vi "模式二.vi"(0 "Input Handle":cluster{"Session":u32, "Card number":u32}, 1 "文件夹路径":path caption="路径", 2 "设置":T1, 5 "error in":errorcluster {"code" format="%.0x"}) -> (14 "Output Handle":cluster{"Session":u32, "Card number":u32}, 19 "error out":errorcluster caption="error in")   [LabVIEW 2018]
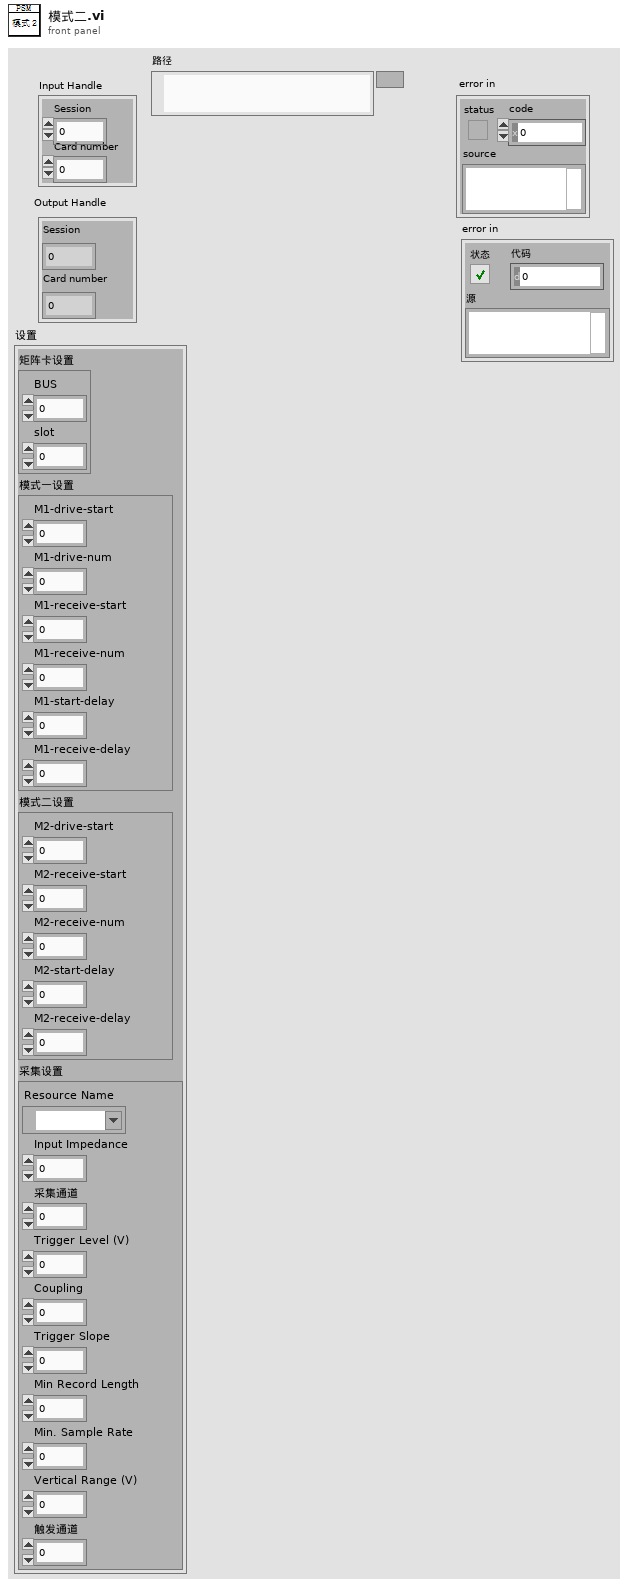
[diagram p1: front panel]
types:
  T1 = cluster{"矩阵卡设置":cluster{"BUS":u32, "slot":u32}, "模式一设置":cluster{"M1-drive-start":u32, "M1-drive-num":u32, "M1-receive-start":u32, "M1-receive-num":u32, "M1-start-delay":u32, "M1-receive-delay":u32}, "模式二设置":cluster{"M2-drive-start":u32, "M2-receive-start":u32, "M2-receive-num":u32, "M2-start-delay":u32, "M2-receive-delay":u32}, "采集设置":cluster{"Resource Name":refnum<k15>, "Input Impedance":u32, "采集通道":i32, "Trigger Level (V)":dbl, "Coupling":u16, "Trigger Slope":i32, "Min Record Length":i32, "Min. Sample Rate":dbl, "Vertical Range (V)":dbl, "触发通道":i32}}
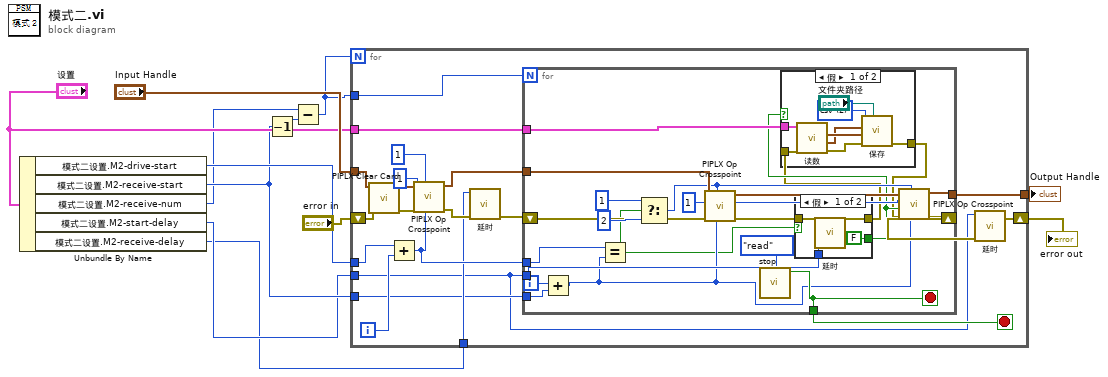
[diagram p0: block diagram]
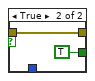
[diagram p3: hidden frame]
diagram:
  n1 = Unbundle By Name("设置") -> ("模式二设置.M2-drive-start"=w5:u32, "模式二设置.M2-receive-start"=w4:u32, "模式二设置.M2-receive-num"=w3:u32, "模式二设置.M2-start-delay"=w2:u32, "模式二设置.M2-receive-delay"=w1:u32)
  n2 = Decrement(x=w4) -> (x-1=w8:u32)
  n3 = Subtract(x=w3, y=w8) -> (x-y=w7:u32)
  n4 = for {
    N: w7 -> [_]
    tunnel: w7 -> [w33]
    tunnel: w5 -> [w30]
    tunnel: "Input Handle" -> [w28]
    tunnel: w2 -> [w14]
    shift-right: [w31] -> w9
    shift-left: "error in" -> [w27]
    tunnel: [w32] -> w10
    tunnel: w1 -> [w16]
    tunnel: w4 -> [w15]
    tunnel: "设置" -> [w13]
    i -> [w29]
    stop <- w20 stop-if-true
    n5 = call <instrlib>:"PIPLX Clear Card.vi"("error in"=w27, "Input Handle"=w28) -> ("error out"=w26:errorcluster, "Output Handle"=w25:cluster{"Session":u32, "Card number":u32})  [unwired: 8 in]
    n6 = Add(x=w30, y=w29) -> (x+y=w21:u32)
    n7 = call <instrlib>:"PIPLX Op Crosspoint.vi"("Column"=w21, "Row"=u32 1, "error in"=w26, "Output Subunit"=u32 1, "Input Handle"=w25) -> ("error out"=w19:errorcluster, "Output Handle"=w24:cluster{"Session":u32, "Card number":u32})  [unwired: 5 in]
    n8 = call "延时.vi"("error in (no error)"=w19, "延时（百毫秒）"=w16) -> ("error out"=w18:errorcluster)  [unwired: 9 in]
    n9 = for {
      N: w33 -> [_]
      tunnel: w21 -> [w53]
      tunnel: w24 -> [w52]
      tunnel: w14 -> [w50]
      shift-right: [w36] -> w17
      shift-left: w18 -> [w51]
      tunnel: [w46] -> w32
      tunnel: [w47] -> w20
      tunnel: w15 -> [w40]
      tunnel: w13 -> [w38]
      i -> [w42]
      stop <- w47 stop-if-true
      w44 = u32 1 ("Output Subunit")
      n10 = Add(x=w42, y=w40) -> (x+y=w41:u32)
      n11 = Equal?(x=w53, y=w41) -> (x = y?=w39:bool)
      n12 = Select(t=u32 1 ("Row"), s=w39, f=u32 2) -> (s? t:f=w43:u32)
      n13 = call <instrlib>:"PIPLX Op Crosspoint.vi"("Column"=w41, "Row"=w43, "error in"=w51, "Output Subunit"=w44, "Input Handle"=w52) -> ("error out"=w49:errorcluster, "Output Handle"=w45:cluster{"Session":u32, "Card number":u32})  [unwired: 5 in]
      n14 = call "stop.vi"("枚举"=enum16{"write", "read"}."read") -> ("停止"=w47:bool)  [unwired: 10 in]
      n15 = case shown="假" w39 {
        tunnel: w50 -> [w68 _]
        tunnel: w49 -> [w67 w70]
        tunnel: [w66 w70] -> w34
        tunnel: [FALSE ("Action") TRUE ("Action")] -> w37
        frame False {
          n16 = call "延时.vi"("error in (no error)"=w67, "延时（百毫秒）"=w68) -> ("error out"=w66:errorcluster)  [unwired: 9 in]
        }
        frame True {
        }
      }
      n17 = case shown="假" w37 {
        tunnel: w34 -> [w56 w64]
        tunnel: [w60 w64] -> w35
        tunnel: w38 -> [w59 _]
        frame False {
          w58 = u16 2 items=["txt", "xls", "csv", "xlsx"] ("文件类型")
          n18 = call "读数.vi"("error in"=w56, "设置"=w59) -> ("error out"=w61:errorcluster, "响应信号"=w62:waveform(dbl), "触发信号"=w63:waveform(dbl))  [unwired: 7 in]
          n19 = call "保存.vi"("文件夹路径"="文件夹路径", "error in (no error)"=w61, "激励信号"=w63, "采集信号"=w62, "文件类型"=w58) -> ("error out"=w60:errorcluster)  [unwired: 6 in]
        }
        frame True {
        }
      }
      n20 = call <instrlib>:"PIPLX Op Crosspoint.vi"("Column"=w41, "Row"=w43, "error in"=w35, "Action"=w37, "Output Subunit"=w44, "Input Handle"=w45) -> ("error out"=w36:errorcluster, "Output Handle"=w46:cluster{"Session":u32, "Card number":u32})  [unwired: 4 in]
    }
    n21 = call "延时.vi"("error in (no error)"=w17, "延时（百毫秒）"=w14) -> ("error out"=w31:errorcluster)  [unwired: 9 in]
  }
  "Output Handle" <- w10
  "error out" <- w9
